vi "set_ocp.vi"(7 "command delay (ms)":u32=100, 8 "error in (no error)":errorcluster, 9 "OCP (V)":dbl, 10 "Channel":string="1", 11 "VISA Refnum in":refnum<visa-resource-name>) -> (0 "error out":errorcluster, 3 "VISA Refnum out":refnum<visa-resource-name>)   [LabVIEW 2018]
panel:
  out "concatenated string":string
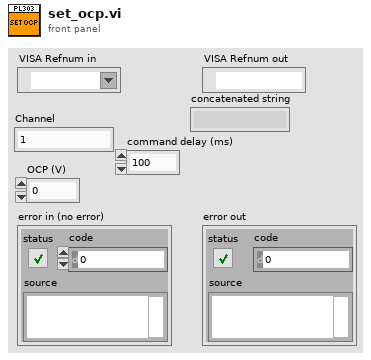
[diagram p1: front panel]
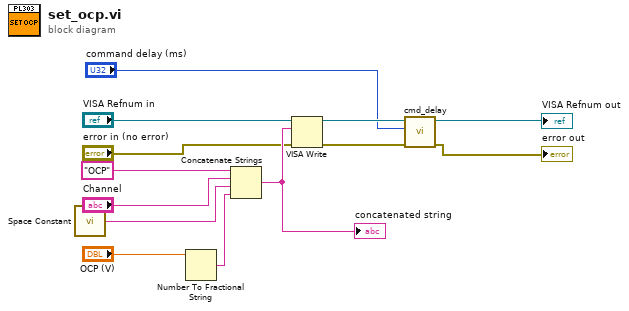
[diagram p0: block diagram]
diagram:
  n1 = call <vilib>:"Space Constant.vi"() -> ("String"=w8:string)
  n2 = Number To Fractional String(number="OCP (V)") -> (F-format string=w6:string)  [unwired: 3 in]
  n3 = Concatenate Strings("OCP" ("string"), "Channel", w8, w6) -> (w11:string)
  "concatenated string" <- w11
  n4 = VISA Write(VISA resource name="VISA Refnum in", write buffer=w11, error in (no error)="error in (no error)") -> (VISA resource name out=w5:refnum<visa-resource-name>, error out=w4:errorcluster)  [unwired: 1 out]
  n5 = call "cmd_delay.vi"("error in (no error)"=w4, "command delay (ms)"="command delay (ms)", "VISA Refnum in"=w5) -> ("error out"=→"error out":errorcluster, "VISA Refnum out"=→"VISA Refnum out":refnum<visa-resource-name>)  [unwired: 7 in]
